vi "Get Serializer.vi"(8 "error in (no error)":errorcluster, 11 "MQTT_Base":refnum<class "MQTT_Base.lvclass">) -> (0 "error out":errorcluster, 2 "Serializer":refnum<class "Serializer.lvclass">, 3 "MQTT_Base out":refnum<class "MQTT_Base.lvclass">)   [LabVIEW 2013, in "MQTT Server.lvlib" / "MQTT_Base.lvclass"]
uses:
  MQTT_Base.lvclass
  <vilib>/LabVIEW Open Source Project/Serializer/Serializer/Serializer.lvclass
  MQTT_Base.lvclass/MQTT_Base.ctl
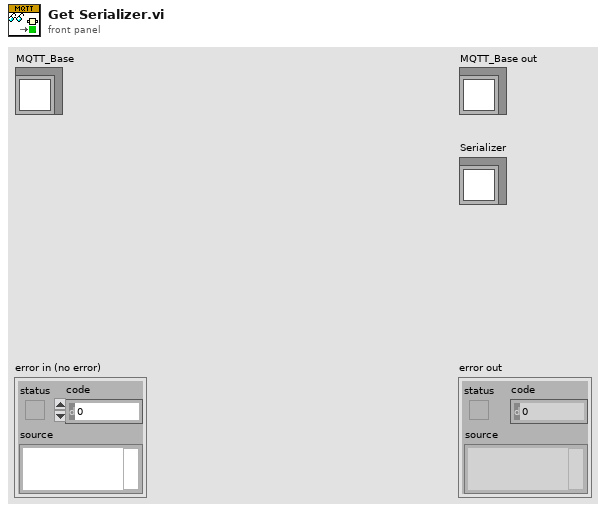
[diagram p1: front panel]
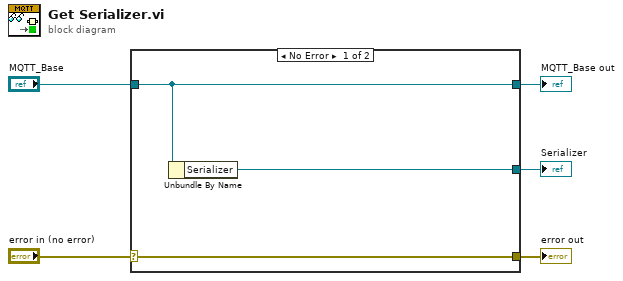
[diagram p0: block diagram]
diagram:
  n1 = case shown="No Error" "error in (no error)" {
    selector: "error in (no error)" -> [w8 w9]
    tunnel: [w8 w9] -> w4
    tunnel: [w7 w10] -> w2
    tunnel: "MQTT_Base" -> [w7 w10]
    tunnel: [w6 _] -> w1
    frame No Error {
      n2 = Unbundle By Name(w7) -> ("Serializer"=w6:refnum<class "Serializer.lvclass">)
    }
    frame Error {
    }
  }
  "error out" <- w4
  "MQTT_Base out" <- w2
  "Serializer" <- w1
